vi "4155C START single v2.0.vi"(4 "error in (no error)":errorcluster, 5 "Emergency Stop":refnum<vi>, 7 "VISA resource name in":refnum<visa-resource-name>) -> (0 "error out":errorcluster, 3 "VISA Resource Name out":refnum<visa-resource-name>)   [LabVIEW 2016]
uses:
  Select Event Type.ctl
panel:
  in  "event resource class":refnum<visa-resource-name>
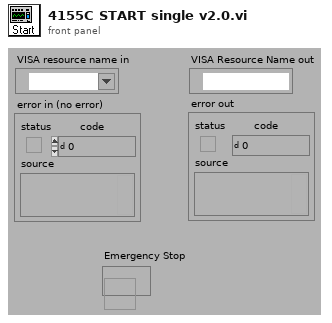
[diagram p1: front panel]
types:
  T1 = typedef "Select Event Type.ctl" = u32
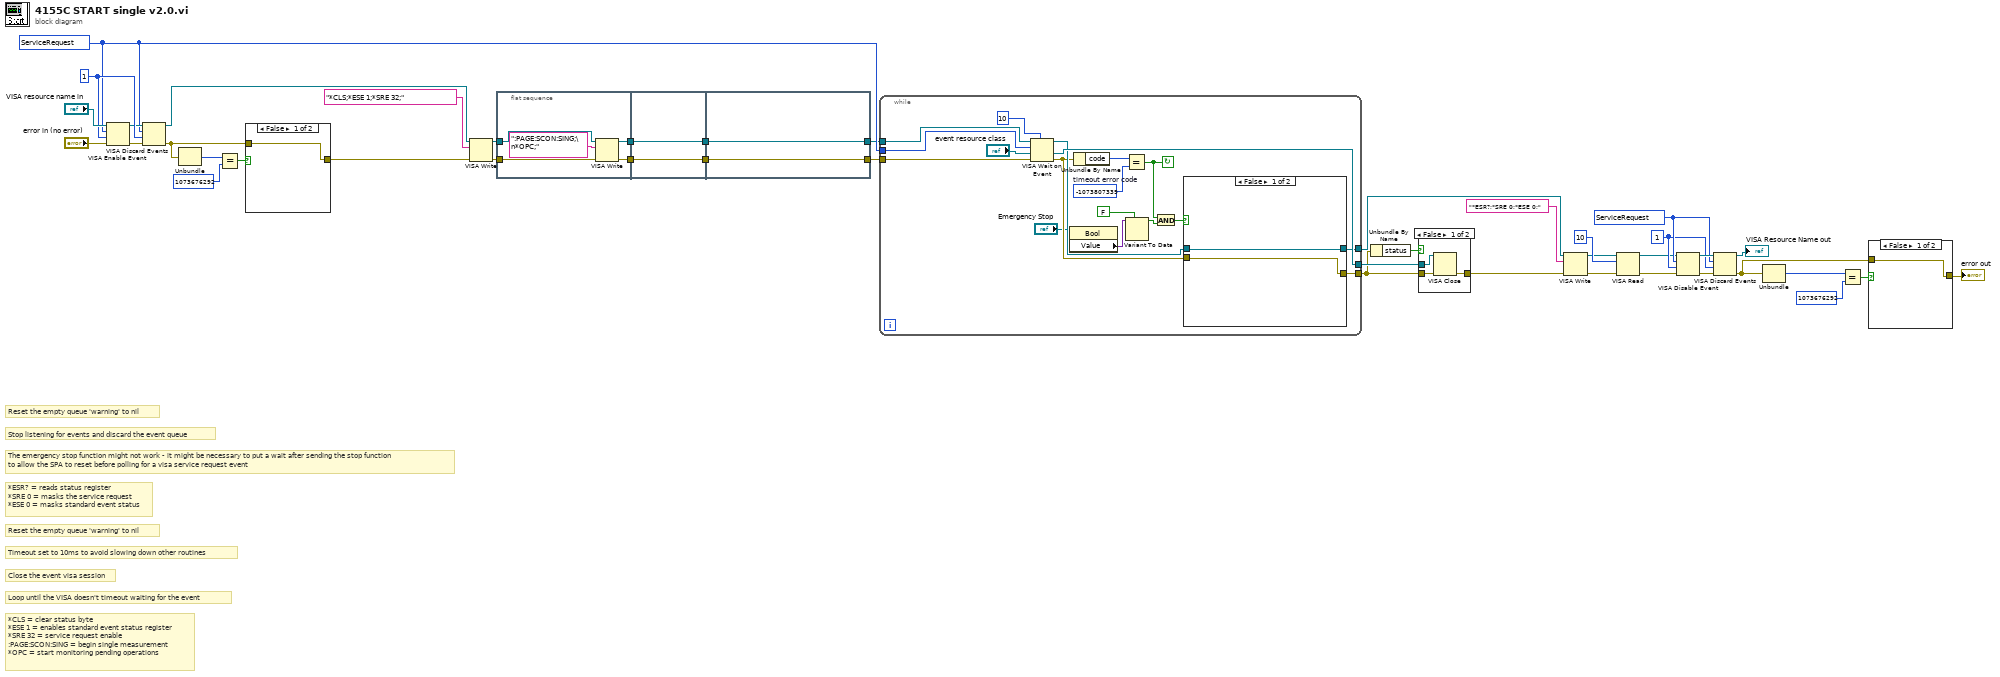
[diagram p0: block diagram]
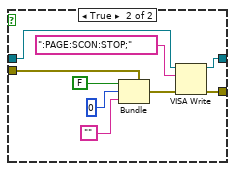
[diagram p2: hidden frame]
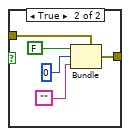
[diagram p3: hidden frame]
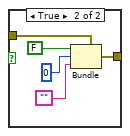
[diagram p4: hidden frame]
diagram:
  w26 = u16 1
  w27 = T1 1073684491 items=["ServiceRequest"=1073684491, "Trigger"=3221168138, "Clear"=1073684493, "VXI-Signal"=1073684512, "VXI/VME-Interrupt"=3221168161, "VXI/VME-Sysfail"=1073684509, "VXI/VME-Sysreset"=1073684510, "GPIB-CIC"=1073684498, "GPIB-Talk"=1073684499, "GPIB-Listen"=1073684500, "PXI-Interrupt"=1073684514, "AllEnabled"=1073709055]
  w35 = T1 1073684491 items=["ServiceRequest"=1073684491, "Trigger"=3221168138, "Clear"=1073684493, "VXI-Signal"=1073684512, "VXI/VME-Interrupt"=3221168161, "VXI/VME-Sysfail"=1073684509, "VXI/VME-Sysreset"=1073684510, "GPIB-CIC"=1073684498, "GPIB-Talk"=1073684499, "GPIB-Listen"=1073684500, "PXI-Interrupt"=1073684514, "AllEnabled"=1073709055] ("Event Type")
  w39 = u32 1 ("mechanism (1:  VI_QUEUE)")
  # "Reset the empty queue 'warning' to nil"
  # "Stop listening for events and discard the event queue"
  # "The emergency stop function might not work - it might be necessary to put a wait after sending the stop function\nto allow the SPA to reset before polling for a visa service request event"
  # "*ESR? = reads status register\n*SRE 0 = masks the service request\n*ESE 0 = masks standard event status"
  # "Reset the empty queue 'warning' to nil"
  # "Timeout set to 10ms to avoid slowing down other routines"
  # "Close the event visa session"
  # "Loop until the VISA doesn't timeout waiting for the event"
  # "*CLS = clear status byte\n*ESE 1 = enables standard event status register\n*SRE 32 = service request enable\n:PAGE:SCON:SING = begin single measurement\n*OPC = start monitoring pending operations"
  n1 = VISA Enable Event(8:"error in (no error)", 9:w39, 10:w35, 11:"VISA resource name in") -> (0:w40:errorcluster, 3:w38:refnum<visa-resource-name>)
  n2 = VISA Discard Events(8:w40, 9:w39, 10:w35, 11:w38) -> (0:w10:errorcluster, 3:w37:refnum<visa-resource-name>)
  n3 = Unbundle(w10) -> ("code"=w13:i32)  [unwired: 2 out]
  n4 = Equal?(x=w13, y=1073676292) -> (x = y?=w11:bool)
  n5 = case shown="False" w11 {
    tunnel: w10 -> [w43 w48]
    tunnel: [w43 w47] -> w9
    frame False {
    }
    frame True {
      n6 = Bundle(cluster=w48, "status"=FALSE, "code"=0, "source"="") -> (w47:errorcluster)
    }
  }
  n7 = VISA Write(VISA resource name=w37, write buffer="*CLS;*ESE 1;*SRE 32;" ("write buffer (\"\")"), error in (no error)=w9) -> (VISA resource name out=w16:refnum<visa-resource-name>, error out=w17:errorcluster)  [unwired: 1 out]
  n8 = flat-sequence {
    tunnel: w17 -> [w53]
    tunnel: w16 -> [w52]
    tunnel: [w51] -> w4
    tunnel: [w50] -> w2
    tunnel: w4 -> [w55]
    tunnel: [w55] -> w3
    tunnel: w2 -> [w54]
    tunnel: [w54] -> w1
    tunnel: [w56] -> w7
    tunnel: [w57] -> w8
    tunnel: w3 -> [w57]
    tunnel: w1 -> [w56]
    frame #0 {
      n9 = VISA Write(VISA resource name=w52, write buffer=":PAGE:SCON:SING;\n*OPC;" ("write buffer (\"\")"), error in (no error)=w53) -> (VISA resource name out=w51:refnum<visa-resource-name>, error out=w50:errorcluster)  [unwired: 1 out]
    }
    frame #1 {
    }
    frame #2 {
    }
  }
  n10 = while {
    tunnel: [w66] -> w5
    tunnel: [w67] -> w14
    tunnel: [w70] -> w18
    tunnel: w35 -> [w72]
    tunnel: w7 -> [w74]
    tunnel: w8 -> [w75]
    stop <- w62 continue-if-true
    w68 = -1073807339  # timeout error code
    n11 = VISA Wait on Event(7:u32 10 ("timeout (0)"), 8:w74, 9:"event resource class", 10:w72, 11:w75) -> (0:w64:errorcluster, 1:w70:refnum<visa-resource-name>, 3:w65:refnum<visa-resource-name>)  [unwired: 1 out]
    n12 = property class="Bool"(reference="Emergency Stop") -> ("Value"=w60:variant)  [unwired: 1 in, 2 out]
    n13 = Unbundle By Name(w64) -> ("code"=w69:i32)
    n14 = Equal?(x=w69, y=w68) -> (x = y?=w62:bool)
    n15 = Variant To Data(type=FALSE, Variant=w60) -> (data=w59:bool)  [unwired: 1 in, 1 out]
    n16 = And(x=w62, y=w59) -> (x .and. y?=w63:bool)
    n17 = case shown="False" w63 {
      tunnel: w64 -> [w76 w82]
      tunnel: w65 -> [w77 w84]
      tunnel: [w77 w85] -> w66
      tunnel: [w76 w86] -> w67
      frame False {
      }
      frame True {
        n18 = Bundle(cluster=w82, "status"=FALSE, "code"=0, "source"="") -> (w78:errorcluster)
        n19 = VISA Write(VISA resource name=w84, write buffer=":PAGE:SCON:STOP;" ("write buffer (\"\")"), error in (no error)=w78) -> (VISA resource name out=w85:refnum<visa-resource-name>, error out=w86:errorcluster)  [unwired: 1 out]
      }
    }
  }
  n20 = Unbundle By Name(w14) -> ("status"=w34:bool)
  n21 = case shown="False" w34 {
    tunnel: w18 -> [w89 _]
    tunnel: w14 -> [w88 w90]
    tunnel: [w87 w90] -> w6
    frame False {
      n22 = VISA Close(VISA resource name=w89, error in (no error)=w88) -> (error out=w87:errorcluster)
    }
    frame True {
    }
  }
  n23 = VISA Write(VISA resource name=w5, write buffer="*ESR?;*SRE 0;*ESE 0;" ("write buffer (\"\")"), error in (no error)=w6) -> (VISA resource name out=w31:refnum<visa-resource-name>, error out=w30:errorcluster)  [unwired: 1 out]
  n24 = VISA Read(VISA resource name=w31, byte count=u32 10, error in (no error)=w30) -> (VISA resource name out=w21:refnum<visa-resource-name>, error out=w20:errorcluster)  [unwired: 2 out]
  n25 = VISA Disable Event(8:w20, 9:w26, 10:w27, 11:w21) -> (0:w28:errorcluster, 3:w29:refnum<visa-resource-name>)
  n26 = VISA Discard Events(8:w28, 9:w26, 10:w27, 11:w29) -> (0:w22:errorcluster, 3:→"VISA Resource Name out":refnum<visa-resource-name>)
  n27 = Unbundle(w22) -> ("code"=w25:i32)  [unwired: 2 out]
  n28 = Equal?(x=w25, y=1073676292) -> (x = y?=w23:bool)
  n29 = case shown="False" w23 {
    tunnel: w22 -> [w91 w96]
    tunnel: [w91 w95] -> w15
    frame False {
    }
    frame True {
      n30 = Bundle(cluster=w96, "status"=FALSE, "code"=0, "source"="") -> (w95:errorcluster)
    }
  }
  "error out" <- w15
